vi "PlaceRandomSnake.vi"(8 "error in (no error)":errorcluster, 11 "Board in":T2[][](array[typedef])) -> (0 "error out":errorcluster, 2 "Positions out":T1, 3 "Board out":T2[][](array[typedef]))   [LabVIEW 2020]
uses:
  TypeDef/tiles-key-trunct.ctl
  TypeDef/direction.ctl
  <vilib>/numeric/Random Number (Range) I64.vi
  <vilib>/numeric/sub_Random U32.vi
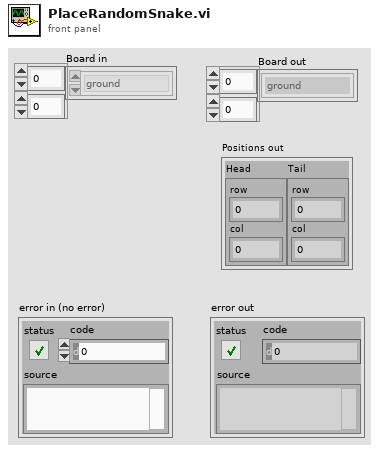
[diagram p1: front panel]
types:
  T1 = cluster{"Head":cluster{"row":i32, "col":i32}, "Tail":cluster{"row":i32, "col":i32}}
  T2 = typedef "tiles-key-trunct.ctl" = enum16{"ground", "wall", "head (right)", "head (up)", "head (left)", "head (down)", "L-turn (right-up)", "L-turn (up-left)", "L-turn (left-down)", "L-turn (down-right)", "body (right)", "body (up)", "body (left)", "body (down)", "R-turn (right-down)", "R-turn (up-right)", "R-turn (left-up)", "R-turn (down-left)", "tail (right)", "tail (up)", "tail (left)", "tail (down)"}
  T3 = typedef "direction.ctl" = enum16{"Right", "Up", "Left", "Down"}
  T4 = cluster{"Direction":T3, "position out":cluster{"row":i32, "col":i32}}
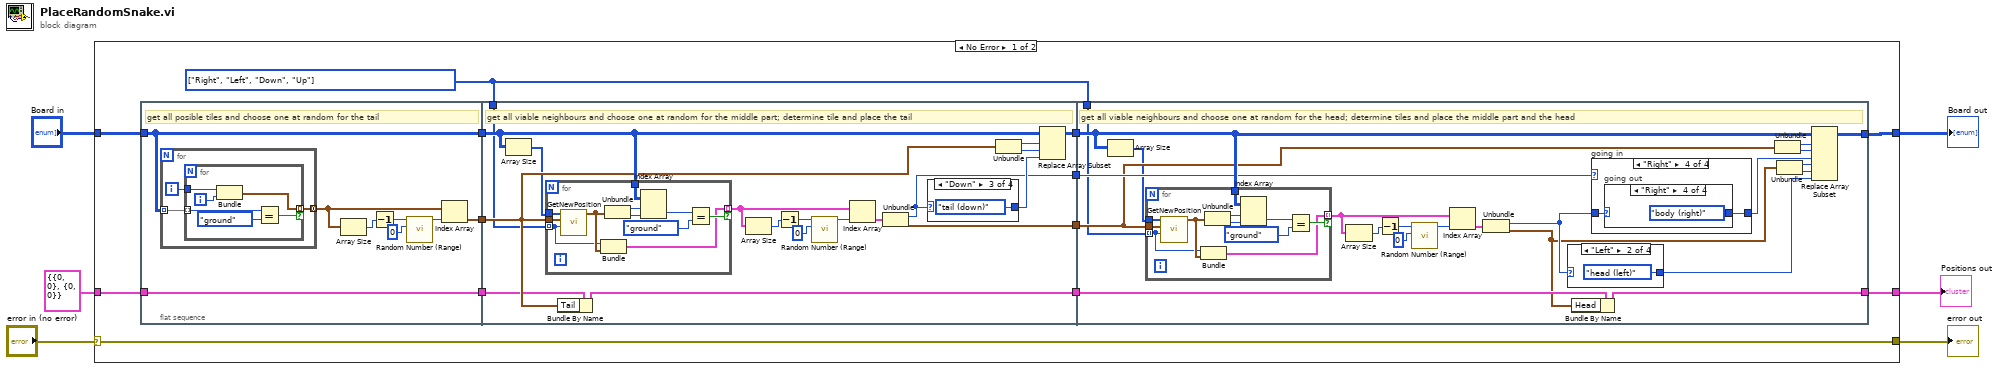
[diagram p0: block diagram]
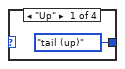
[diagram p2: hidden frame]
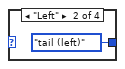
[diagram p3: hidden frame]
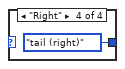
[diagram p4: hidden frame]
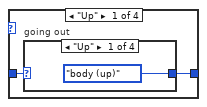
[diagram p5: hidden frame]
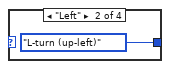
[diagram p6: hidden frame]
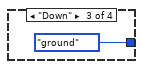
[diagram p7: hidden frame]
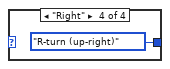
[diagram p8: hidden frame]
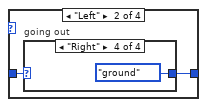
[diagram p9: hidden frame]
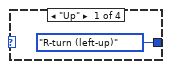
[diagram p10: hidden frame]
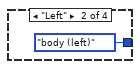
[diagram p11: hidden frame]
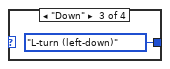
[diagram p12: hidden frame]
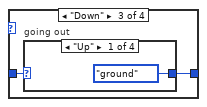
[diagram p13: hidden frame]
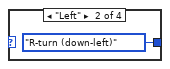
[diagram p14: hidden frame]
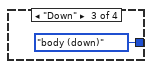
[diagram p15: hidden frame]
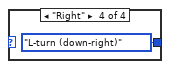
[diagram p16: hidden frame]
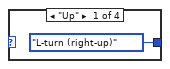
[diagram p17: hidden frame]
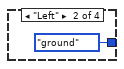
[diagram p18: hidden frame]
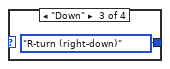
[diagram p19: hidden frame]
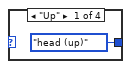
[diagram p20: hidden frame]
diagram:
  n1 = case shown="No Error" "error in (no error)" {
    selector: "error in (no error)" -> [w19 w133]
    tunnel: [w19 w133] -> w5
    tunnel: "Board in" -> [w16 w132]
    tunnel: [w9 w132] -> w3
    tunnel: [w8 w131] -> w2
    tunnel: T1 {"Head"={"row"=0, "col"=0}, "Tail"={"row"=0, "col"=0}} ("Positions out") -> [w7 w131]
    frame No Error {
      w10 = T3[] [enum."Right", enum."Left", enum."Down", enum."Up"] items=["Right", "Up", "Left", "Down"] ("Array")
      n2 = flat-sequence {
        tunnel: [w21] -> w18
        tunnel: [w22] -> w17
        tunnel: w16 -> [w22]
        tunnel: [w20] -> w15
        tunnel: w7 -> [w20]
        tunnel: [w52] -> w14
        tunnel: [w48] -> w13
        tunnel: [w47] -> w12
        tunnel: [w46] -> w11
        tunnel: w15 -> [w37]
        tunnel: w17 -> [w54]
        tunnel: w10 -> [w45]
        tunnel: w18 -> [w51]
        tunnel: [w86] -> w9
        tunnel: [w89] -> w8
        tunnel: w10 -> [w70]
        tunnel: w11 -> [w83]
        tunnel: w12 -> [w88]
        tunnel: w13 -> [w91]
        tunnel: w14 -> [w90]
        frame #0 {
          # "get all posible tiles and choose one at random for the tail"
          n3 = for {
            tunnel: w22 -> [w29] mode=indexing
            tunnel: [w28] -> w27 mode=concatenating
            i -> [w30]
            # "get all possible tiles"
            n4 = for {
              tunnel: w30 -> [w35]
              tunnel: w29 -> [w33] mode=indexing
              tunnel: [w34] -> w28 mode=indexing if=w32
              i -> [w36]
              n5 = Bundle(w35, w36) -> (w34:cluster{i32, i32})  [unwired: 1 in]
              n6 = Equal?(x=w33, y=tiles-key-trunct."ground") -> (x = y?=w32:bool)
            }
          }
          n7 = Array Size(array=w27) -> (size(s)=w25:i32)
          n8 = Decrement(x=w25) -> (x-1=w23:i32)
          n9 = call-poly <vilib>:"Random Number (Range).vi"("lower bound (-100)"=i64 0, "upper bound (100)"=w23) -> ("number"=w26:i64)  [unwired: 9 in]
          n10 = Index Array(array=w27, index=w26) -> (element=w21:cluster{i32, i32})
        }
        frame #1 {
          # "get all viable neighbours and choose one at random for the middle part; determine tile and place the tail"
          n11 = Array Size(array=w54) -> (size(s)=w44:i32[])
          n12 = for {
            tunnel: w44 -> [w65]
            tunnel: w51 -> [w64]
            tunnel: w45 -> [w55] mode=indexing
            tunnel: w54 -> [w63]
            tunnel: [w57] -> w39 mode=indexing if=w58
            n13 = call "GetNewPosition.vi"("Direction"=w55, "position in"=w64, "size(s)"=w65) -> ("position out"=w56:cluster{"row":i32, "col":i32})  [unwired: 8 in]
            n14 = Bundle("Direction"=w55, "position out"=w56) -> (w57:T4)  [unwired: 1 in]
            n15 = Unbundle(w56) -> ("row"=w62:i32, "col"=w61:i32)
            n16 = Index Array(array=w63, index (row)=w62, index (col)=w61) -> (element=w60:T2)
            n17 = Equal?(x=w60, y=tiles-key-trunct."ground") -> (x = y?=w58:bool)
          }
          n18 = Bundle By Name(cluster=w37, "Tail"=w51) -> (w48:T1)
          n19 = Array Size(array=w39) -> (size(s)=w43:i32)
          n20 = Decrement(x=w43) -> (x-1=w41:i32)
          n21 = call-poly <vilib>:"Random Number (Range).vi"("lower bound (-100)"=i64 0, "upper bound (100)"=w41) -> ("number"=w40:i64)  [unwired: 9 in]
          n22 = Index Array(array=w39, index=w40) -> (element=w38:T4)
          n23 = Unbundle(w38) -> ("Direction"=w47:T3, "position out"=w46:cluster{"row":i32, "col":i32})
          n24 = case shown="\"Down\"" w47 {
            tunnel: [tiles-key-trunct."tail (up)" ("y") tiles-key-trunct."tail (left)" ("y") tiles-key-trunct."tail (down)" ("y") tiles-key-trunct."tail (right)" ("y")] -> w53
            frame "Up" {
            }
            frame "Left" {
            }
            frame "Down" {
            }
            frame "Right" {
            }
          }
          n25 = Unbundle(w51) -> (w50:i32, w49:i32)
          n26 = Replace Array Subset(array=w54, new element=w53, index (row)=w50, index (col)=w49) -> (w52:T2[][])
        }
        frame #2 {
          # "get all viable neighbours and choose one at random for the head; determine tiles and place the middle part and the head"
          n27 = Array Size(array=w90) -> (size(s)=w77:i32[])
          n28 = for {
            tunnel: w77 -> [w102]
            tunnel: w83 -> [w101]
            tunnel: w70 -> [w92] mode=indexing
            tunnel: w90 -> [w100]
            tunnel: [w94] -> w72 mode=indexing if=w95
            n29 = call "GetNewPosition.vi"("Direction"=w92, "position in"=w101, "size(s)"=w102) -> ("position out"=w93:cluster{"row":i32, "col":i32})  [unwired: 8 in]
            n30 = Bundle("Direction"=w92, "position out"=w93) -> (w94:T4)  [unwired: 1 in]
            n31 = Unbundle(w93) -> ("row"=w99:i32, "col"=w98:i32)
            n32 = Index Array(array=w100, index (row)=w99, index (col)=w98) -> (element=w97:T2)
            n33 = Equal?(x=w97, y=tiles-key-trunct."ground") -> (x = y?=w95:bool)
          }
          n34 = Array Size(array=w72) -> (size(s)=w76:i32)
          n35 = Decrement(x=w76) -> (x-1=w74:i32)
          n36 = call-poly <vilib>:"Random Number (Range).vi"("lower bound (-100)"=i64 0, "upper bound (100)"=w74) -> ("number"=w73:i64)  [unwired: 9 in]
          n37 = Index Array(array=w72, index=w73) -> (element=w71:T4)
          n38 = Unbundle(w71) -> ("Direction"=w87:T3, "position out"=w80:cluster{"row":i32, "col":i32})
          n39 = case shown="\"Left\"" w87 {
            tunnel: [tiles-key-trunct."head (up)" ("y") tiles-key-trunct."head (left)" ("y") tiles-key-trunct."head (down)" ("y") tiles-key-trunct."head (right)" ("y")] -> w84
            frame "Up" {
            }
            frame "Left" {
            }
            frame "Down" {
            }
            frame "Right" {
            }
          }
          n40 = Bundle By Name(cluster=w91, "Head"=w80) -> (w89:T1)
          n41 = case "going in" shown="\"Right\"" w88 {
            tunnel: w87 -> [w104 w110 w116 w122]
            tunnel: [w103 w109 w115 w121] -> w85
            frame "Up" {
              # "in"
              n42 = case "going out" shown="\"Up\"" w104 {
                tunnel: [tiles-key-trunct."body (up)" ("y") tiles-key-trunct."L-turn (up-left)" ("y") tiles-key-trunct."ground" ("y") tiles-key-trunct."R-turn (up-right)" ("y")] -> w103
                frame "Up" {
                }
                frame "Left" {
                }
                frame "Down" {
                }
                frame "Right" {
                }
              }
            }
            frame "Left" {
              # "in"
              n43 = case "going out" shown="\"Right\"" w110 {
                tunnel: [tiles-key-trunct."R-turn (left-up)" ("y") tiles-key-trunct."body (left)" ("y") tiles-key-trunct."L-turn (left-down)" ("y") tiles-key-trunct."ground" ("y")] -> w109
                frame "Up" {
                }
                frame "Left" {
                }
                frame "Down" {
                }
                frame "Right" {
                }
              }
            }
            frame "Down" {
              # "in"
              n44 = case "going out" shown="\"Up\"" w116 {
                tunnel: [tiles-key-trunct."ground" ("y") tiles-key-trunct."R-turn (down-left)" ("y") tiles-key-trunct."body (down)" ("y") tiles-key-trunct."L-turn (down-right)" ("y")] -> w115
                frame "Up" {
                }
                frame "Left" {
                }
                frame "Down" {
                }
                frame "Right" {
                }
              }
            }
            frame "Right" {
              # "in"
              n45 = case "going out" shown="\"Right\"" w122 {
                tunnel: [tiles-key-trunct."L-turn (right-up)" ("y") tiles-key-trunct."ground" ("y") tiles-key-trunct."R-turn (right-down)" ("y") tiles-key-trunct."body (right)" ("y")] -> w121
                frame "Up" {
                }
                frame "Left" {
                }
                frame "Down" {
                }
                frame "Right" {
                }
              }
            }
          }
          n46 = Unbundle(w83) -> ("row"=w82:i32, "col"=w81:i32)
          n47 = Unbundle(w80) -> ("row"=w79:i32, "col"=w78:i32)
          n48 = Replace Array Subset(array=w90, new element #1=w85, index (row) #1=w82, index (col) #1=w81, new element #2=w84, index (row) #2=w79, index (col) #2=w78) -> (w86:T2[][])
        }
      }
    }
    frame Error {
    }
  }
  "Board out" <- w3
  "Positions out" <- w2
  "error out" <- w5
